vi "calc T and P.vi"(7 "DAQ cluster in":T1 {"temp"."utility"."therm volt" format="%_6g"; "temp"."utility"."heat volt in" format="%_6g"; "temp"."utility"."heat volt out" format="%_6g"; "temp"."utility"."power out" format="%_6g"; "temp"."utility"."H Vmax" format="%_6g"; "temp"."T exec"."man power" format="%_6g"; "temp"."T exec"."exec setpoint" format="%_6g"; "temp"."T params"."Settle Time" step=1.0; "temp"."T params"."Settle Bandwidth" step=0.01; "temp"."T params"."Derivative Tme" step=0.01; "temp"."T params"."Integral Time" step=1.0; "temp"."T params"."Control Bandwidth" step=0.1; "temp"."T params"."Setpoint" step=0.1; "temp"."T status"."Setpoint" format="%_6g"; "temp"."T status"."Power" format="%_6g"; "temp"."T status"."Temp" format="%_6g"}) -> (8 "DAQ cluster out":T1 {"temp"."utility"."therm volt" format="%_6g"; "temp"."utility"."heat volt in" format="%_6g"; "temp"."utility"."heat volt out" format="%_6g"; "temp"."utility"."power out" format="%_6g"; "temp"."utility"."H Vmax" format="%_6g"; "temp"."T exec"."man power" format="%_6g"; "temp"."T exec"."exec setpoint" format="%_6g"; "temp"."T params"."Settle Time" step=1.0; "temp"."T params"."Settle Bandwidth" step=0.01; "temp"."T params"."Derivative Tme" step=0.01; "temp"."T params"."Integral Time" step=1.0; "temp"."T params"."Control Bandwidth" step=0.1; "temp"."T params"."Setpoint" step=0.1; "temp"."T status"."Setpoint" format="%_6g"; "temp"."T status"."Power" format="%_6g"; "temp"."T status"."Temp" format="%_6g"})   [LabVIEW 2019]
doc: "This subVI is a component of the meas T and P state of the DAQ state machine in the bug experiment.\n\nThis subVI calculates the current time, the bug temerature, and the bug heater power from the raw voltage measurements and saves the data to arunning array for graphing.\n\nIt records the history of the time, temperature, and power.\nIt also logs the temp control parameters is logging is active.\n\nPaul K Dixon\nP3600\nCSUSB Physics"
uses:
  typedefs/DAQ state cluster.ctl
  typedefs/DAQ state enum.ctl
  typedefs/temp cont cluster.ctl
  typedefs/temp exec cluster.ctl
  typedefs/temp mode enum.ctl
  typedefs/temp indicator.ctl
  typedefs/temp control status.ctl
  typedefs/PID control parameters.ctl
  typedefs/temp cont utility.ctl
  typedefs/measurement.ctl
  typedefs/wvfm acq params.ctl
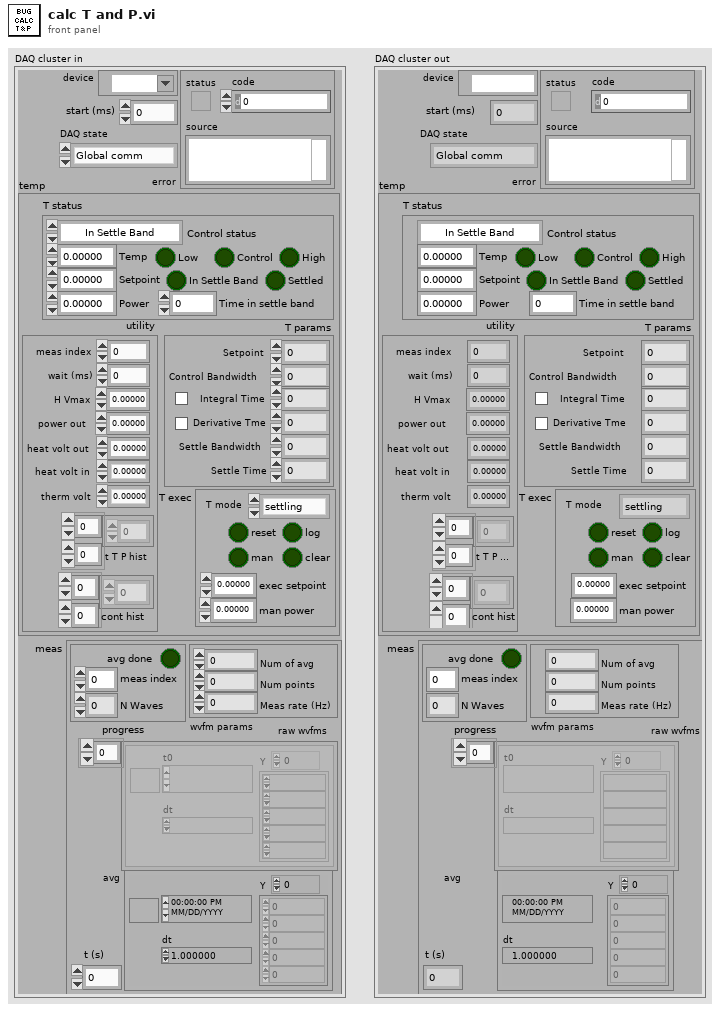
[diagram p1: front panel]
types:
  T1 = typedef "DAQ state cluster.ctl" = cluster{"DAQ state":T2, "temp":T3, "meas":T10, "device":tag, "error":errorcluster, "start (ms)":i32}
  T2 = typedef "DAQ state enum.ctl" = enum16{"Global comm", "Meas T & P", "PID power calc", "Man Power set", "Output Power", "Wait", "Meas wvfm", "Avg wvfm", "Exit"}
  T3 = typedef "temp cont cluster.ctl" = cluster{"T exec":T4, "T status":T6, "T params":T8, "utility":T9}
  T4 = typedef "temp exec cluster.ctl" = cluster{"T mode":T5, "exec setpoint":dbl, "reset":bool, "man power":dbl, "man":bool, "log":bool, "clear":bool}
  T5 = typedef "temp mode enum.ctl" = enum16{"settling", "measuring", "holding", "Exit"}
  T6 = typedef "temp indicator.ctl" = cluster{"Control status":T7, "Temp":dbl, "Power":dbl, "Time in settle band":dbl, "Settled":bool, "Low":bool, "High":bool, "Setpoint":dbl, "Control":bool, "In Settle Band":bool}
  T7 = typedef "temp control status.ctl" = enum16{"In Settle Band", "In Control Band", "Below Control Band", "Above Control Band"}
  T8 = typedef "PID control parameters.ctl" = cluster{"Setpoint":dbl, "Control Bandwidth":dbl, "Integral Time":dbl, "Int\nON":bool, "Derivative Tme":dbl, "Der\nON":bool, "Settle Bandwidth":dbl, "Settle Time":dbl}
  T9 = typedef "temp cont utility.ctl" = cluster{"meas index":i32, "wait (ms)":i32, "H Vmax":dbl, "power out":dbl, "heat volt out":dbl, "heat volt in":dbl, "therm volt":dbl, "t T P hist":dbl[][], "cont hist":dbl[][]}
  T10 = typedef "measurement.ctl" = cluster{"wvfm params":T11, "avg":waveform(dbl), "raw wvfms":waveform(dbl)[], "progress":cluster{"avg done":bool, "meas index":i32, "N waves":i32}, "t (s)":dbl}
  T11 = typedef "wvfm acq params.ctl" = cluster{"Num of avg":i32, "Num points":i32, "Meas rate (Hz)":dbl}
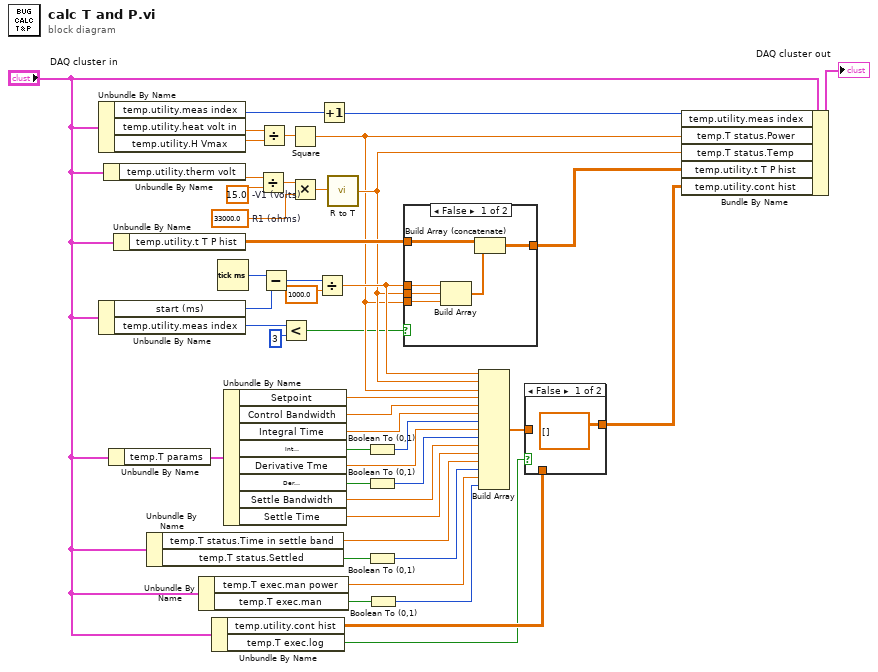
[diagram p0: block diagram]
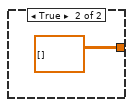
[diagram p2: hidden frame]
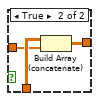
[diagram p3: hidden frame]
diagram:
  w40 = 15.0  # -V1 (volts)
  w38 = 33000.0  # R1 (ohms)
  n1 = Unbundle By Name("DAQ cluster in") -> ("temp.utility.meas index"=w6:i32, "temp.utility.heat volt in"=w44:dbl, "temp.utility.H Vmax"=w43:dbl)
  n2 = Unbundle By Name("DAQ cluster in") -> ("start (ms)"=w34:i32, "temp.utility.meas index"=w3:i32)
  n3 = Unbundle By Name("DAQ cluster in") -> ("temp.utility.therm volt"=w41:dbl)
  n4 = Unbundle By Name("DAQ cluster in") -> ("temp.T params"=w21:T8)
  n5 = Unbundle By Name("DAQ cluster in") -> ("temp.utility.t T P hist"=w36:dbl[][])
  n6 = Unbundle By Name("DAQ cluster in") -> ("temp.T status.Time in settle band"=w19:dbl, "temp.T status.Settled"=w20:bool)
  n7 = Unbundle By Name("DAQ cluster in") -> ("temp.T exec.man power"=w13:dbl, "temp.T exec.man"=w14:bool)
  n8 = Unbundle By Name("DAQ cluster in") -> ("temp.utility.cont hist"=w17:dbl[][], "temp.T exec.log"=w15:bool)
  n9 = Tick Count (ms)() -> (millisecond timer value=w35:u32)
  n10 = Unbundle By Name(w21) -> ("Setpoint"=w24:dbl, "Control Bandwidth"=w25:dbl, "Integral Time"=w26:dbl, "Int\nON"=w27:bool, "Derivative Tme"=w30:dbl, "Der\nON"=w28:bool, "Settle Bandwidth"=w23:dbl, "Settle Time"=w22:dbl)
  n11 = Divide(x=w41, y=w40) -> (x/y=w39:dbl)
  n12 = Divide(x=w44, y=w43) -> (x/y=w42:dbl)
  n13 = Subtract(x=w35, y=w34) -> (x-y=w33:u32)
  n14 = Less?(x=w3, y=3) -> (x < y?=w1:bool)
  n15 = Square(x=w42) -> (x^2=w7:dbl)
  n16 = Multiply(x=w39, y=w38) -> (x*y=w37:dbl)
  n17 = Divide(x=w33, y=1000.0) -> (x/y=w10:dbl)
  n18 = Increment(x=w6) -> (x+1=w5:i32)
  n19 = call "R to T.vi"("Resistance (Ohm)"=w37) -> ("Temp (deg C)"=w9:dbl)  [unwired: 13 in, 1 out]
  n20 = Boolean To (0,1)(Boolean=w27) -> (0, 1=w29:i16)
  n21 = Boolean To (0,1)(Boolean=w28) -> (0, 1=w31:i16)
  n22 = Boolean To (0,1)(Boolean=w20) -> (0, 1=w18:i16)
  n23 = Boolean To (0,1)(Boolean=w14) -> (0, 1=w12:i16)
  n24 = case shown="False" w1 {
    tunnel: w36 -> [w51 _]
    tunnel: w10 -> [w50 _]
    tunnel: w9 -> [w49 _]
    tunnel: w7 -> [w47 _]
    tunnel: [w46 dbl[][] []] -> w4
    frame False {
      n25 = Build Array(w50, w49, w47) -> (w48:dbl[])
      n26 = Build Array (concatenate)(w51, w48) -> (w46:dbl[][])
    }
    frame True {
    }
  }
  n27 = Build Array(w10, w9, w7, w24, w25, w26, w29, w30, w31, w23, w22, w19, w18, w13, w12) -> (w16:dbl[])
  n28 = case shown="False" w15 {
    tunnel: w17 -> [_ w56]
    tunnel: w16 -> [_ w55]
    tunnel: [dbl[][] [] w54] -> w8
    frame False {
    }
    frame True {
      n29 = Build Array (concatenate)(w56, w55) -> (w54:dbl[][])
    }
  }
  n30 = Bundle By Name(cluster="DAQ cluster in", "temp.utility.meas index"=w5, "temp.T status.Power"=w7, "temp.T status.Temp"=w9, "temp.utility.t T P hist"=w4, "temp.utility.cont hist"=w8) -> (→"DAQ cluster out":T1)
